vi "Test 4.vi"() -> ()   [LabVIEW 2019]
panel:
  out "已强制转换(x)":dbl
  out "范围内？":bool
  in  "x":dbl
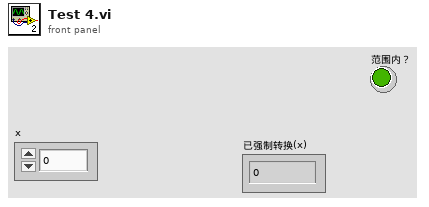
[diagram p1: front panel]
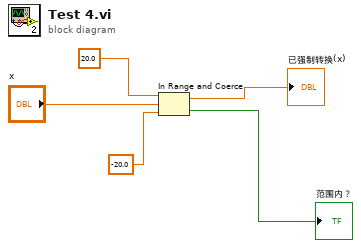
[diagram p0: block diagram]
diagram:
  n1 = In Range and Coerce(upper limit=20.0 ("上限"), x="x", lower limit=-20.0 ("下限")) -> (coerced(x)=→"已强制转换(x)":dbl, In Range?=→"范围内？":bool)
